vi "change control params.vi"(7 "exp exec in":errorcluster) -> (8 "exp exec in":errorcluster)   [LabVIEW 2019]
doc: "Used as a popup subvi to allow the user to modify the current temperature control parameters.\n\nThe setpoint is part of the list for convenience, but not actionable. It's value is controlled by the executive setpoint instead; it is ovewrwritten is soon at the user finished editing the parameters and returns to execution via proceed.\n\nPaul K Dixon\nPhysics 350\nCSUSB Physics"
uses:
  typedefs/PID control parameters.ctl
  globals/Bug globals.vi
panel:
  in  "Cancel Button":bool
  in  "OK Button":bool
  in  "Control Parameters":T1={"Setpoint"=30.0, "Control Bandwidth"=4.0, "Integral Time"=20.0, "Int\nON"=TRUE, "Derivative Tme"=0.4, "Der\nON"=TRUE, "Settle Bandwidth"=0.20000000000000007, "Settle Time"=60.0} {"Settle Time" step=1.0; "Settle Bandwidth" step=0.01; "Derivative Tme" step=0.01; "Integral Time" step=1.0; "Control Bandwidth" step=0.1; "Setpoint" step=0.1}
  # "Note:\nThe setpoint is controlled\nseperately\n\nthis instance is overwritten\nby the executive setpoint"
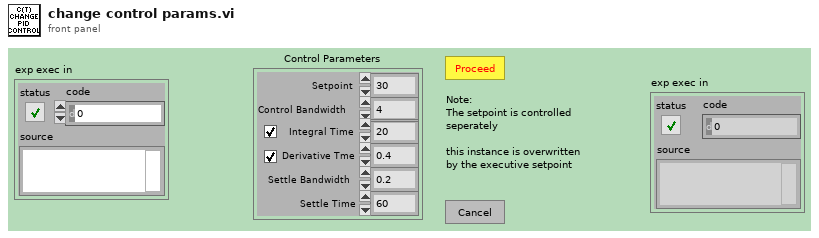
[diagram p1: front panel]
types:
  T1 = typedef "PID control parameters.ctl" = cluster{"Setpoint":dbl, "Control Bandwidth":dbl, "Integral Time":dbl, "Int\nON":bool, "Derivative Tme":dbl, "Der\nON":bool, "Settle Bandwidth":dbl, "Settle Time":dbl}
  T2 = typedef "temp cont cluster.ctl" = cluster{"T exec":T3, "T status":T5, "T params":T1, "utility":T7}
  T3 = typedef "temp exec cluster.ctl" = cluster{"T mode":T4, "exec setpoint":dbl, "reset":bool, "man power":dbl, "man":bool, "log":bool, "clear":bool}
  T4 = typedef "temp mode enum.ctl" = enum16{"settling", "measuring", "holding", "Exit"}
  T5 = typedef "temp indicator.ctl" = cluster{"Control status":T6, "Temp":dbl, "Power":dbl, "Time in settle band":dbl, "Settled":bool, "Low":bool, "High":bool, "Setpoint":dbl, "Control":bool, "In Settle Band":bool}
  T6 = typedef "temp control status.ctl" = enum16{"In Settle Band", "In Control Band", "Below Control Band", "Above Control Band"}
  T7 = typedef "temp cont utility.ctl" = cluster{"meas index":i32, "wait (ms)":i32, "H Vmax":dbl, "power out":dbl, "heat volt out":dbl, "heat volt in":dbl, "therm volt":dbl, "t T P hist":dbl[][], "cont hist":dbl[][]}
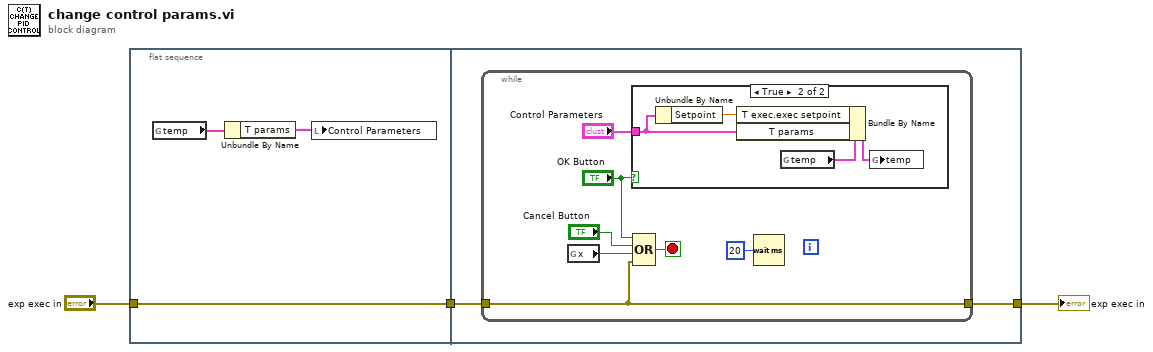
[diagram p0: block diagram]
diagram:
  n1 = flat-sequence {
    tunnel: [w4] -> w1
    tunnel: "exp exec in" -> [w4]
    tunnel: w1 -> [w8]
    tunnel: [w7] -> w3
    frame #0 {
      n2 = global read "Bug globals.vi" "temp"() -> (w6:T2)
      n3 = Unbundle By Name(w6) -> ("T params"=w5:T1)
      n4 = local write "Control Parameters"(w5) -> ()
    }
    frame #1 {
      n5 = while {
        tunnel: w8 -> [w10]
        tunnel: [w10] -> w7
        stop <- w15 stop-if-true
        n6 = global read "Bug globals.vi" "x"() -> (w9:bool)
        n7 = case shown="True" "OK Button" {
          tunnel: "Control Parameters" -> [_ w17]
          frame False {
          }
          frame True {
            n8 = Unbundle By Name(w17) -> ("Setpoint"=w16:dbl)
            n9 = global read "Bug globals.vi" "temp"() -> (w19:T2)
            n10 = Bundle By Name(cluster=w19, "T exec.exec setpoint"=w16, "T params"=w17) -> (w18:T2)
            n11 = global write "Bug globals.vi" "temp"(w18) -> ()
          }
        }
        n12 = Compound Arithmetic op=OR("OK Button", "Cancel Button", w9, w10) -> (w15:bool)
        n13 = Wait (ms)(milliseconds to wait=u32 20) -> ()  [unwired: 1 out]
      }
    }
  }
  "exp exec in" <- w3
